vi "Ramp SRS 830 output V.vi"() -> ()   [LabVIEW 2024]
panel:
  in  "STOP 2":bool
  out "Current Value 2":dbl
  in  "Set Point 2":dbl min=-10.0 max=10.0 step=0.1 format="%.3f"
  in  "Rate V/S 2":dbl=0.00167 min=-1.0 max=1.0 step=0.0001 format="%_3e"
  out "Current Value":dbl
  in  "Set Point":dbl min=-10.0 max=10.0 step=0.1 format="%.3f"
  in  "STOP":bool
  in  "Rate V/S":dbl=0.00167 min=-1.0 max=1.0 step=0.0001 format="%_3e"
  in  "GPIB Address":refnum<visa-resource-name>
  # "Channel 1"
  # "Channel 2"
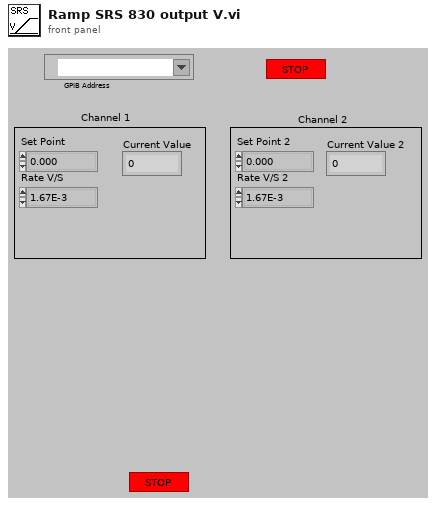
[diagram p1: front panel]
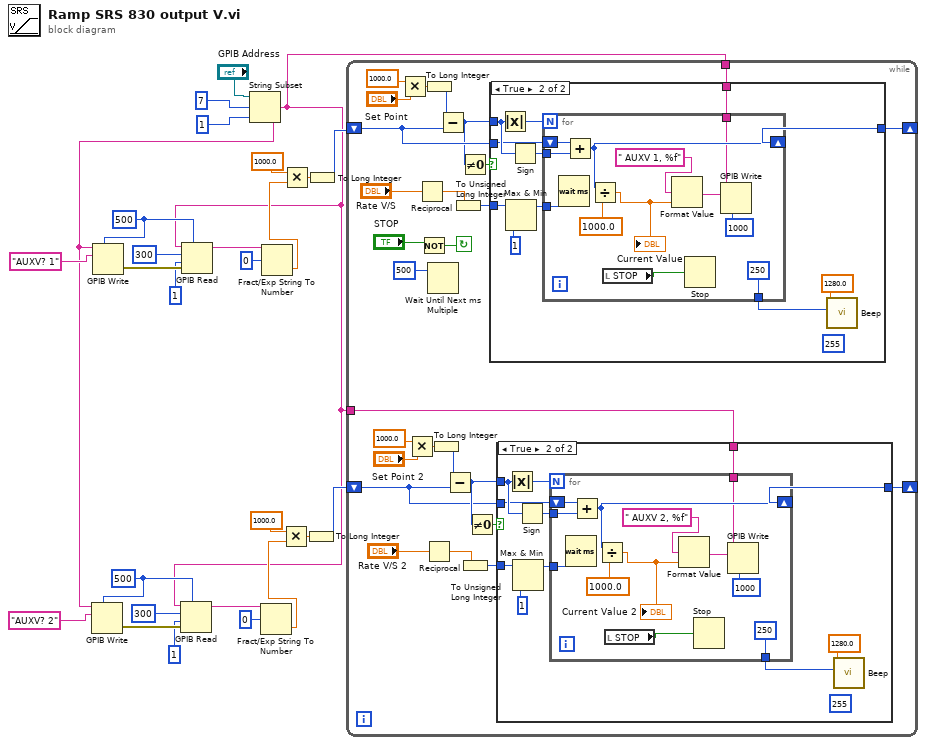
[diagram p0: block diagram]
diagram:
  w10 = 500 ("timeout ms (488.2 global)")
  w20 = 500 ("timeout ms (488.2 global)")
  n1 = String Subset(string="GPIB Address", offset (0)=7, length (rest)=1 ("length (rest)")) -> (substring=w1:string)
  n2 = GPIB Write(0:w1, 1:"AUXV? 2" ("string"), 4:w10) -> (6:w9:errorcluster)  [unwired: 2 in, 1 out]
  n3 = GPIB Write(0:w1, 1:"AUXV? 1" ("string"), 4:w20) -> (6:w19:errorcluster)  [unwired: 2 in, 1 out]
  n4 = GPIB Read(0:w1, 1:300 ("byte count"), 2:i16 1 ("mode (0)"), 3:w9, 4:w10) -> (5:w6:string)  [unwired: 2 out]
  n5 = GPIB Read(0:w1, 1:300 ("byte count"), 2:i16 1 ("mode (0)"), 3:w19, 4:w20) -> (5:w16:string)  [unwired: 2 out]
  n6 = Fract/Exp String To Number(string=w6, offset=0) -> (number=w4:dbl)  [unwired: 2 in, 1 out]
  n7 = Fract/Exp String To Number(string=w16, offset=0) -> (number=w14:dbl)  [unwired: 2 in, 1 out]
  n8 = Multiply(x=1000.0, y=w4) -> (x*y=w11:dbl)
  n9 = Multiply(x=1000.0, y=w14) -> (x*y=w25:dbl)
  n10 = To Long Integer(number=w11) -> (32bit integer=w2:i32)
  n11 = To Long Integer(number=w25) -> (32bit integer=w24:i32)
  n12 = while {
    shift-left: w24 -> [w49]
    shift-right: [w50] -> _
    tunnel: w1 -> [w40]
    shift-right: [w28] -> _
    shift-left: w2 -> [w29]
    tunnel: w1 -> [w27]
    stop <- w52 continue-if-true
    n13 = Multiply(x=1000.0, y="Set Point") -> (x*y=w43:dbl)
    n14 = Multiply(x=1000.0, y="Set Point 2") -> (x*y=w33:dbl)
    n15 = Reciprocal(x="Rate V/S") -> (1/x=w51:dbl)
    n16 = Not(x="STOP") -> (.not. x?=w52:bool)
    n17 = To Long Integer(number=w43) -> (32bit integer=w41:i32)
    n18 = Reciprocal(x="Rate V/S 2") -> (1/x=w38:dbl)
    n19 = Wait Until Next ms Multiple(millisecond multiple=u32 500) -> ()  [unwired: 1 out]
    n20 = To Long Integer(number=w33) -> (32bit integer=w31:i32)
    n21 = Subtract(x=w41, y=w49) -> (x-y=w47:i32)
    n22 = Subtract(x=w31, y=w29) -> (x-y=w36:i32)
    n23 = To Unsigned Long Integer(number=w51) -> (unsigned 32bit integer=w48:u32)
    n24 = Not Equal To 0?(x=w47) -> (x != 0?=w46:bool)
    n25 = To Unsigned Long Integer(number=w38) -> (unsigned 32bit integer=w37:u32)
    n26 = Not Equal To 0?(x=w36) -> (x != 0?=w35:bool)
    n27 = case shown="True" w46 {
      tunnel: w48 -> [_ w86]
      tunnel: w49 -> [w78 w87]
      tunnel: w47 -> [_ w88]
      tunnel: [w78 w89] -> w50
      tunnel: w40 -> [_ w79]
      frame False {
      }
      frame True {
        (unwired) i16 255
        n28 = Absolute Value(x=w88) -> (abs(x)=w84:i32)
        n29 = Max & Min(x=w86, y=1) -> (max(x,y)=w83:u32)  [unwired: 1 out]
        n30 = Sign(1:w88) -> (0:w85:i32)
        n31 = for {
          N: w84 -> [_]
          shift-right: [w94] -> w89
          shift-left: w87 -> [w98]
          tunnel: w83 -> [w97]
          tunnel: w85 -> [w99]
          tunnel: [i16 250] -> w80
          tunnel: w79 -> [w92]
          n32 = Wait (ms)(milliseconds to wait=w97) -> ()  [unwired: 1 out]
          n33 = Add(x=w98, y=w99) -> (x+y=w94:i32)
          n34 = Divide(x=w94, y=1000.0) -> (x/y=w95:dbl)
          "Current Value" <- w95
          n35 = local read "STOP"() -> (w90:bool)
          n36 = Format Value(format string=" AUXV 1, %f", value (0)=w95) -> (output string=w100:string)  [unwired: 1 in]
          n37 = Stop(stop? (T)=w90) -> ()
          n38 = GPIB Write(0:w92, 1:w100, 4:1000) -> ()  [unwired: 2 in, 2 out]
        }
        n39 = call <vilib>:"Beep.vi"("duration (msec)"=w80, "frequency (Hz)"=1280.0) -> ()  [unwired: 10 in]
      }
    }
    n40 = case shown="True" w35 {
      tunnel: w37 -> [_ w62]
      tunnel: w29 -> [w54 w63]
      tunnel: w36 -> [_ w64]
      tunnel: [w54 w65] -> w28
      tunnel: w27 -> [_ w55]
      frame False {
      }
      frame True {
        (unwired) i16 255
        n41 = Absolute Value(x=w64) -> (abs(x)=w60:i32)
        n42 = Max & Min(x=w62, y=1) -> (max(x,y)=w59:u32)  [unwired: 1 out]
        n43 = Sign(1:w64) -> (0:w61:i32)
        n44 = for {
          N: w60 -> [_]
          shift-right: [w70] -> w65
          shift-left: w63 -> [w74]
          tunnel: w59 -> [w73]
          tunnel: w61 -> [w75]
          tunnel: [i16 250] -> w56
          tunnel: w55 -> [w68]
          n45 = Wait (ms)(milliseconds to wait=w73) -> ()  [unwired: 1 out]
          n46 = Add(x=w74, y=w75) -> (x+y=w70:i32)
          n47 = Divide(x=w70, y=1000.0) -> (x/y=w71:dbl)
          "Current Value 2" <- w71
          n48 = local read "STOP"() -> (w66:bool)
          n49 = Format Value(format string=" AUXV 2, %f", value (0)=w71) -> (output string=w76:string)  [unwired: 1 in]
          n50 = Stop(stop? (T)=w66) -> ()
          n51 = GPIB Write(0:w68, 1:w76, 4:1000) -> ()  [unwired: 2 in, 2 out]
        }
        n52 = call <vilib>:"Beep.vi"("duration (msec)"=w56, "frequency (Hz)"=1280.0) -> ()  [unwired: 10 in]
      }
    }
  }
